vi "VI Transform Wrapper.vi"(8 "error in (no error)":errorcluster, 11 "Value in (1,-1)":dbl) -> (0 "error out":errorcluster, 3 "Value out (-1,1)":dbl)   [LabVIEW 2012]
doc: "If we have already encountered an error, this VI will do nothing. Otherwise, this VI will take an input, coerce it to be in range and then use a table lookup to determine the scaled value."
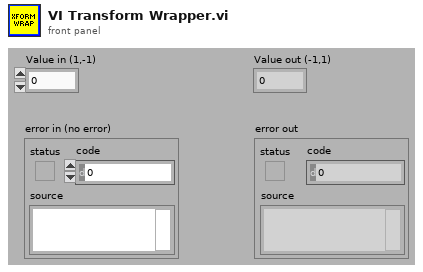
[diagram p1: front panel]
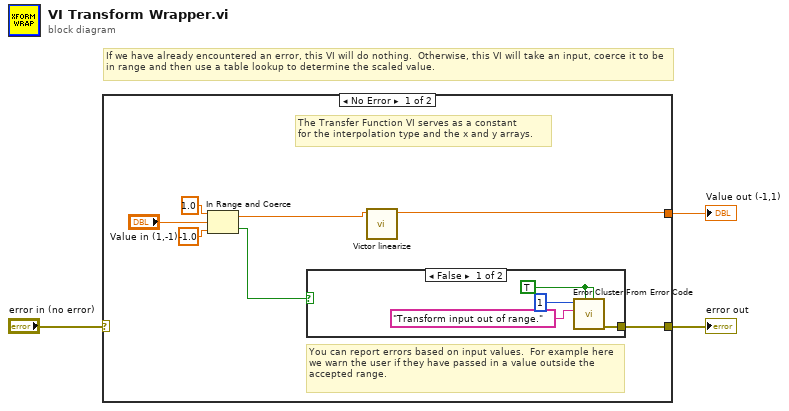
[diagram p0: block diagram]
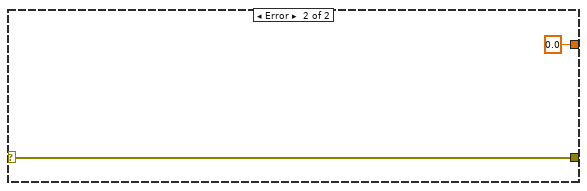
[diagram p3: hidden frame]
diagram:
  # "If we have already encountered an error, this VI will do nothing.  Otherwise, this VI will take an input, coerce it to be in range and then use a table lookup to determine the scaled value."
  n1 = case shown="No Error" "error in (no error)" {
    selector: "error in (no error)" -> [_ w16]
    tunnel: [w7 w16] -> w2
    tunnel: [w4 0.0 ("Output")] -> w1
    frame No Error {
      # "The Transfer Function VI serves as a constant \nfor the interpolation type and the x and y arrays."
      # "You can report errors based on input values.  For example here we warn the user if they have passed in a value outside the accepted range."
      n2 = In Range and Coerce(upper limit=1.0, x="Value in (1,-1)", lower limit=-1.0) -> (coerced(x)=w5:dbl, In Range?=w6:bool)
      n3 = case shown="False" w6 {
        tunnel: [w11 _] -> w7
        frame False {
          w14 = TRUE ("show call chain? (False)")
          n4 = call <vilib>:"Error Cluster From Error Code.vi"("is warning? (False)"=w14, "show call chain? (False)"=w14, "error message (\"\")"="Transform input out of range." ("error message (\"\")"), "error code (0)"=1) -> ("error out"=w11:errorcluster)  [unwired: 1 in, 4 out]
        }
        frame True {
        }
      }
      n5 = call "Victor linearize.vi"("Input"=w5) -> ("Output"=w4:dbl)  [unwired: 10 in]
    }
    frame Error {
    }
  }
  "error out" <- w2
  "Value out (-1,1)" <- w1
